vi "Database.CheckExist.vi"(7 "Idx":i32, 8 "error in":errorcluster, 9 "Serial":string, 10 "Ref":string, 11 "Data in":T1) -> (0 "error out":errorcluster, 2 "Exist":bool, 3 "Data out":T1)   [LabVIEW 2016]
uses:
  Cache/Cache.SystemID.Fglb.Action.ctl
  Database.Data.Sets.ctl
  Database.Data.Status.ctl
  Database.Data.ctl
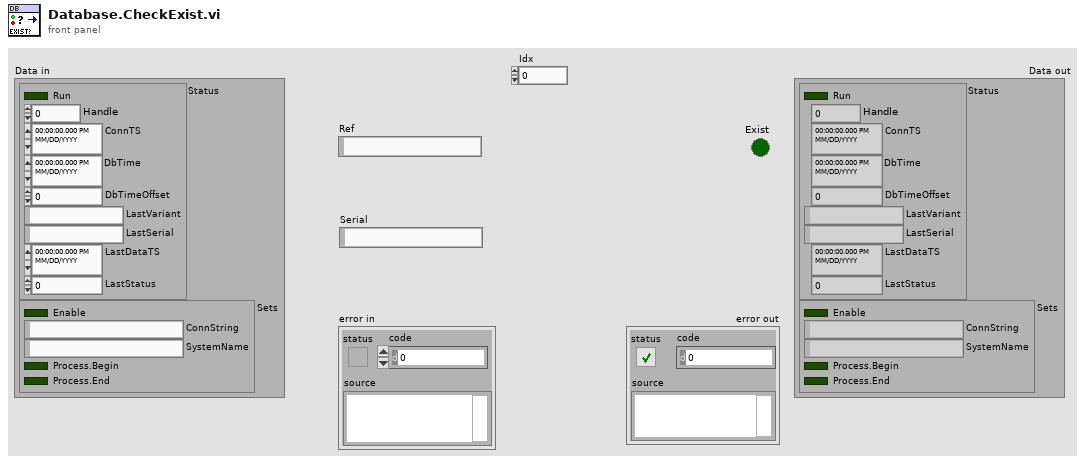
[diagram p1: front panel]
types:
  T1 = typedef "Database.Data.ctl" = cluster{"Status":T2, "Sets":T3}
  T2 = typedef "Database.Data.Status.ctl" = cluster{"Run":bool, "Handle":i32, "ConnTS":timestamp, "DbTime":timestamp, "DbTimeOffset":dbl, "LastVariant":string, "LastSerial":string, "LastDataTS":timestamp, "LastStatus":i32}
  T3 = typedef "Database.Data.Sets.ctl" = cluster{"Enable":bool, "ConnString":string, "SystemName":string, "Process.Begin":bool, "Process.End":bool}
  T4 = typedef "Cache.SystemID.Fglb.Action.ctl" = enum16{"init", "add", "add CheckExistSystem", "add PrevSystem", "get", "get CheckExistSystem", "get PrevSystem"}
  T5 = typedef "ProdaNG.Identification.ctl" = cluster{"processId":i32, "systemId":i32, "processStepId":i32, "wabcoPartId":i32}
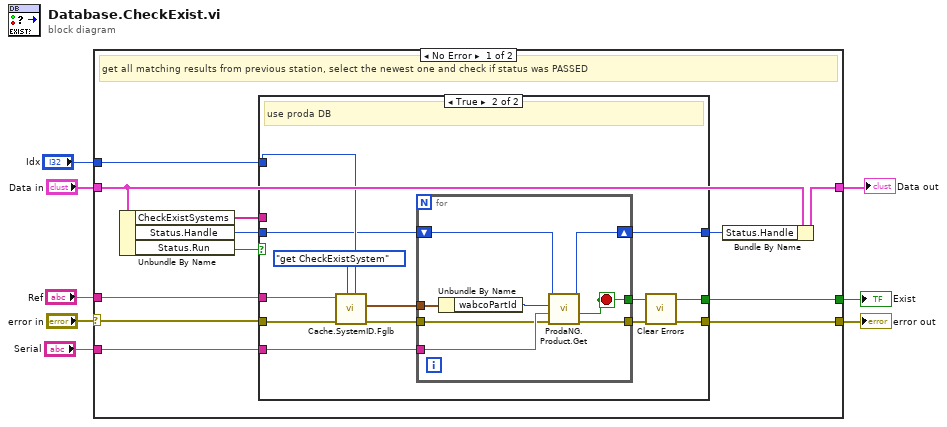
[diagram p0: block diagram]
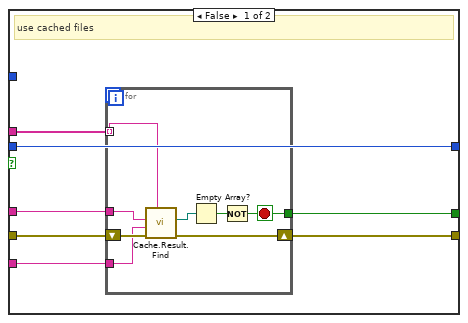
[diagram p2: hidden frame]
diagram:
  n1 = case shown="No Error" "error in" {
    selector: "error in" -> [w19 w57]
    tunnel: [w20 w57] -> w8
    tunnel: [w9 _] -> w6
    tunnel: "Data in" -> [w16 w56]
    tunnel: [w15 w56] -> w4
    tunnel: "Ref" -> [w12 _]
    tunnel: "Idx" -> [w11 _]
    tunnel: "Serial" -> [w10 _]
    frame No Error {
      # "get all matching results from previous station, select the newest one and check if status was PASSED"
      n2 = Unbundle By Name(w16) -> ("CheckExistSystems"=w18:string[], "Status.Handle"=w17:i32, "Status.Run"=w13:bool)
      n3 = case shown="True" w13 {
        tunnel: w19 -> [w26 w44]
        tunnel: [w23 w36] -> w20
        tunnel: w10 -> [w24 w46]
        tunnel: w18 -> [w21 _]
        tunnel: w17 -> [w27 w40]
        tunnel: [w27 w45] -> w14
        tunnel: w12 -> [w25 w43]
        tunnel: w11 -> [_ w42]
        tunnel: [w22 w37] -> w9
        frame False {
          # "use cached files"
          n4 = for {
            tunnel: w25 -> [w34]
            tunnel: w24 -> [w32]
            shift-right: [w33] -> w23
            shift-left: w26 -> [w35]
            tunnel: w21 -> [w31] mode=indexing
            tunnel: [w28] -> w22
            stop <- w28 stop-if-true
            n5 = call "Cache.Result.Find.vi"("Idx"=w31, "error in (no error)"=w35, "Serial"=w32, "Variant"=w34) -> ("error out"=w33:errorcluster, "File"=w29:path)  [unwired: 5 in, 1 out]
            n6 = Empty Array?(array=w29) -> (empty?=w30:bool)
            n7 = Not(x=w30) -> (.not. x?=w28:bool)
          }
        }
        frame True {
          # "use proda DB"
          n8 = call "Cache.SystemID.Fglb.vi"("Station"=w42, "Action (get)"=Cache.SystemID.Fglb.Action."get CheckExistSystem", "error in (no error)"=w44, "Variant"=w43) -> ("error out"=w41:errorcluster, "SytemID"=w38:T5)  [unwired: 5 in, 1 out]
          n9 = for {
            tunnel: w46 -> [w55]
            shift-right: [w49] -> w45
            shift-left: w40 -> [w52]
            tunnel: w38 -> [w51]
            tunnel: [w48] -> w37
            tunnel: w41 -> [w53]
            tunnel: [w50] -> w47
            stop <- w48 stop-if-true
            n10 = Unbundle By Name(w51) -> ("wabcoPartId"=w54:i32)
            n11 = call "ProdaNG.Product.Get.vi"("error in (no error)"=w53, "serialNumber"=w55, "wabcoPartId"=w54, "dbHandle"=w52) -> ("error out"=w50:errorcluster, "found"=w48:bool, "dbHandle out"=w49:i32)  [unwired: 4 in, 1 out]
          }
          n12 = call <vilib>:"Clear Errors.vi"("error in (no error)"=w47) -> ("error out"=w36:errorcluster)  [unwired: 5 in, 1 out]
        }
      }
      n13 = Bundle By Name(cluster=w16, "Status.Handle"=w14) -> (w15:T1)
    }
    frame Error {
    }
  }
  "error out" <- w8
  "Exist" <- w6
  "Data out" <- w4
